vi "WPI_IMU_ADIS16448_WriteRegister.vi"(8 "error in":errorcluster, 9 "Data":u16 format="%x", 10 "Address":u16 format="%x", 11 "SPIDevRef in":T1={"DevStatus"={"status"=FALSE, "code"=0, "source"=""}, "Handle"=0, "Controller"=enum."Controller 1", "SPI Bus"=enum."Invalid"}) -> (0 "error out":errorcluster, 3 "SPIDevRef out":T1)   [LabVIEW 2014, in "ADIS16448.lvlib"]
uses:
  ADIS16448.lvlib
  <vilib>/Rock Robotics/WPI/SPI/WPI_SPIDevRef.ctl
  <vilib>/Rock Robotics/SystemInterfaces/Typedef/FPGA_TypedefDigitalModule.ctl
  <vilib>/Rock Robotics/SystemInterfaces/spilib/spi_bus.ctl
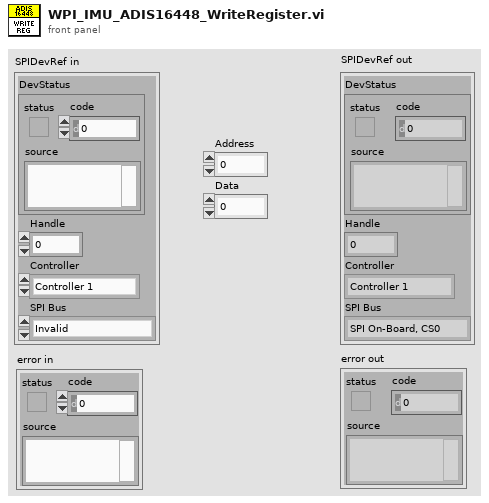
[diagram p1: front panel]
types:
  T1 = typedef "WPI_SPIDevRef.ctl" = cluster{"DevStatus":errorcluster, "Handle":i32, "Controller":T2, "SPI Bus":T3}
  T2 = typedef "FPGA_TypedefDigitalModule.ctl" = enum16{"Controller 1"}
  T3 = typedef "spi_bus.ctl" = enum16{"SPI On-Board, CS0", "SPI On-Board, CS1", "SPI On-Board, CS2", "SPI On-Board, CS3", "SPI MXP", "Invalid"}
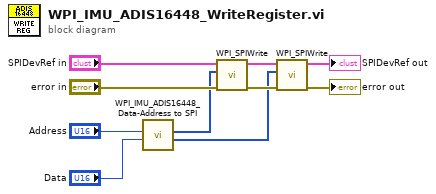
[diagram p0: block diagram]
diagram:
  n1 = call "WPI_IMU_ADIS16448_Data-Address to SPI.vi"("Data"="Data", "Address"="Address") -> ("Low Word"=w3:u8[], "High Word"=w4:u8[])  [unwired: 8 in]
  n2 = call <vilib>:"WPI_SPIWrite.vi"("error in (no error)"="error in", "Data To Send"=w4, "SPIDevRef"="SPIDevRef in") -> ("error out"=w7:errorcluster, "SPIDevRef"=w9:T1)  [unwired: 6 in, 1 out]
  n3 = call <vilib>:"WPI_SPIWrite.vi"("error in (no error)"=w7, "Data To Send"=w3, "SPIDevRef"=w9) -> ("error out"=→"error out":errorcluster, "SPIDevRef"=→"SPIDevRef out":T1)  [unwired: 6 in, 1 out]
